vi "sub_vi_uarv7.vi"(8 "error in (no error)":errorcluster, 11 "Queue in":refnum<queue>) -> (0 "error out":errorcluster, 3 "queue out":refnum<queue>)   [LabVIEW 2023]
uses:
  perionica_states.ctl
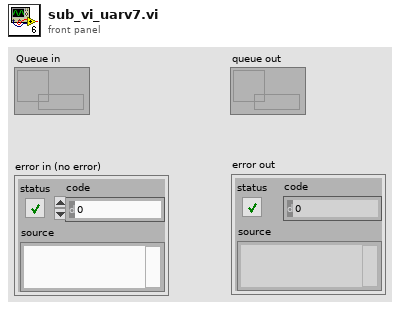
[diagram p1: front panel]
types:
  T1 = typedef "perionica_states.ctl" = enum16{"Zaustavljeno", "Pranje sasije", "Samponiranje", "Voskiranje", "Ispiranje", "Susenje"}
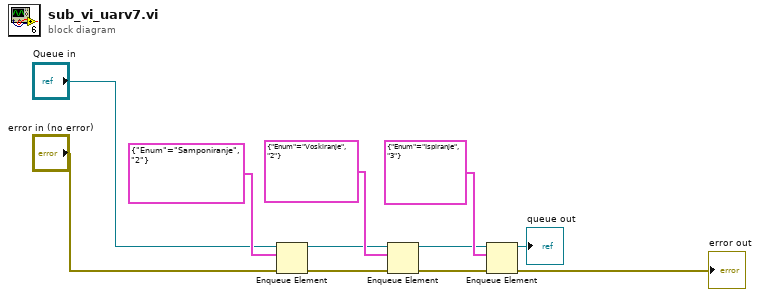
[diagram p0: block diagram]
diagram:
  n1 = Enqueue Element(queue="Queue in", element=cluster{"Enum":T1, string} {"Enum"=enum."Samponiranje", "2"}, error in (no error)="error in (no error)") -> (queue out=w7:refnum<queue>, error out=w6:errorcluster)  [unwired: 1 in, 1 out]
  n2 = Enqueue Element(queue=w7, element=cluster{"Enum":T1, string} {"Enum"=enum."Voskiranje", "2"}, error in (no error)=w6) -> (queue out=w10:refnum<queue>, error out=w9:errorcluster)  [unwired: 1 in, 1 out]
  n3 = Enqueue Element(queue=w10, element=cluster{"Enum":T1, string} {"Enum"=enum."Ispiranje", "3"}, error in (no error)=w9) -> (queue out=→"queue out":refnum<queue>, error out=→"error out":errorcluster)  [unwired: 1 in, 1 out]
